vi "AutoCAD busy 64bit.vi"(6 "error in (no error)":errorcluster, 7 "Application":refnum<k7>) -> (2 "error out":errorcluster, 3 "IsQuiescent":bool)   [LabVIEW 2011, in "Design Server.lvlib"]
uses:
  Design Server.lvlib
panel:
  out "Numeric":i32
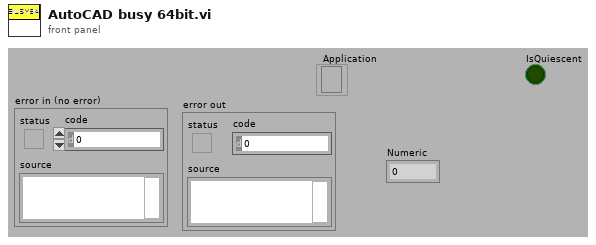
[diagram p1: front panel]
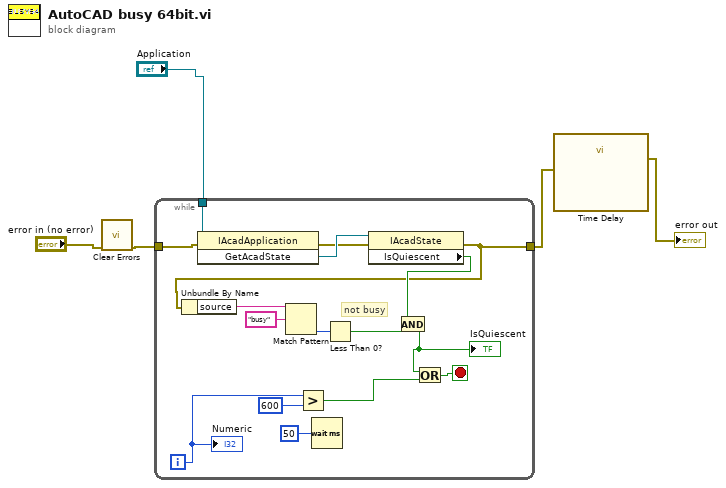
[diagram p0: block diagram]
diagram:
  n1 = call <vilib>:"Clear Errors.vi"("error in (no error)"="error in (no error)") -> ("error out"=w4:errorcluster)  [unwired: 6 in]
  n2 = while {
    tunnel: "Application" -> [w11]
    tunnel: w4 -> [w10]
    tunnel: [w6] -> w3
    i -> [w18]
    stop <- w17 stop-if-true
    # "not busy"
    n3 = invoke class="IAcadApplication" method="GetAcadState"(reference=w11, error in=w10) -> (error out=w8:errorcluster, "GetAcadState"=w9:refnum<k7>)  [unwired: 1 in, 1 out]
    n4 = Greater?(x=w18, y=600) -> (0:w20:bool)
    n5 = Wait (ms)(milliseconds to wait=u32 50) -> ()  [unwired: 1 out]
    n6 = property class="IAcadState"(reference=w9, error in=w8) -> (error out=w6:errorcluster, "IsQuiescent"=w7:bool)  [unwired: 1 out]
    n7 = Unbundle By Name(w6) -> ("source"=w16:string)
    n8 = Match Pattern(string=w16, regular expression="busy") -> (offset past match=w14:i32)  [unwired: 1 in, 3 out]
    n9 = Less Than 0?(x=w14) -> (x < 0?=w13:bool)
    n10 = And(x=w7, y=w13) -> (x .and. y?=w12:bool)
    "IsQuiescent" <- w12
    n11 = Or(x=w12, y=w20) -> (x .or. y?=w17:bool)
    "Numeric" <- w18
  }
  n12 = call "Time Delay"("error in (no error)"=w3) -> ("error out"=→"error out":errorcluster)  [unwired: 10 in]
